vi "Update Method Event Unbundlers.vi"(8 "error in (no error)":errorcluster, 11 "VI ref in":refnum<vi>) -> (0 "error out":errorcluster, 2 "RPC Method Name":string, 3 "VI ref out":refnum<vi>)   [LabVIEW 2019, in "gRPC Scripting Tools.lvlib"]
uses:
  gRPC Scripting Tools.lvlib
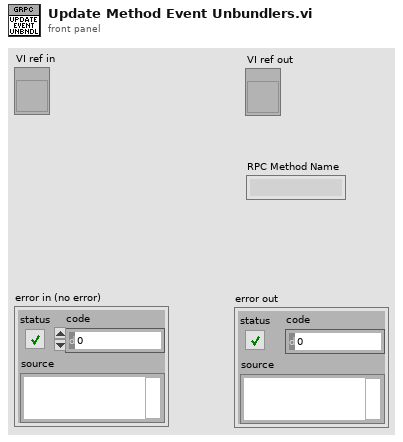
[diagram p1: front panel]
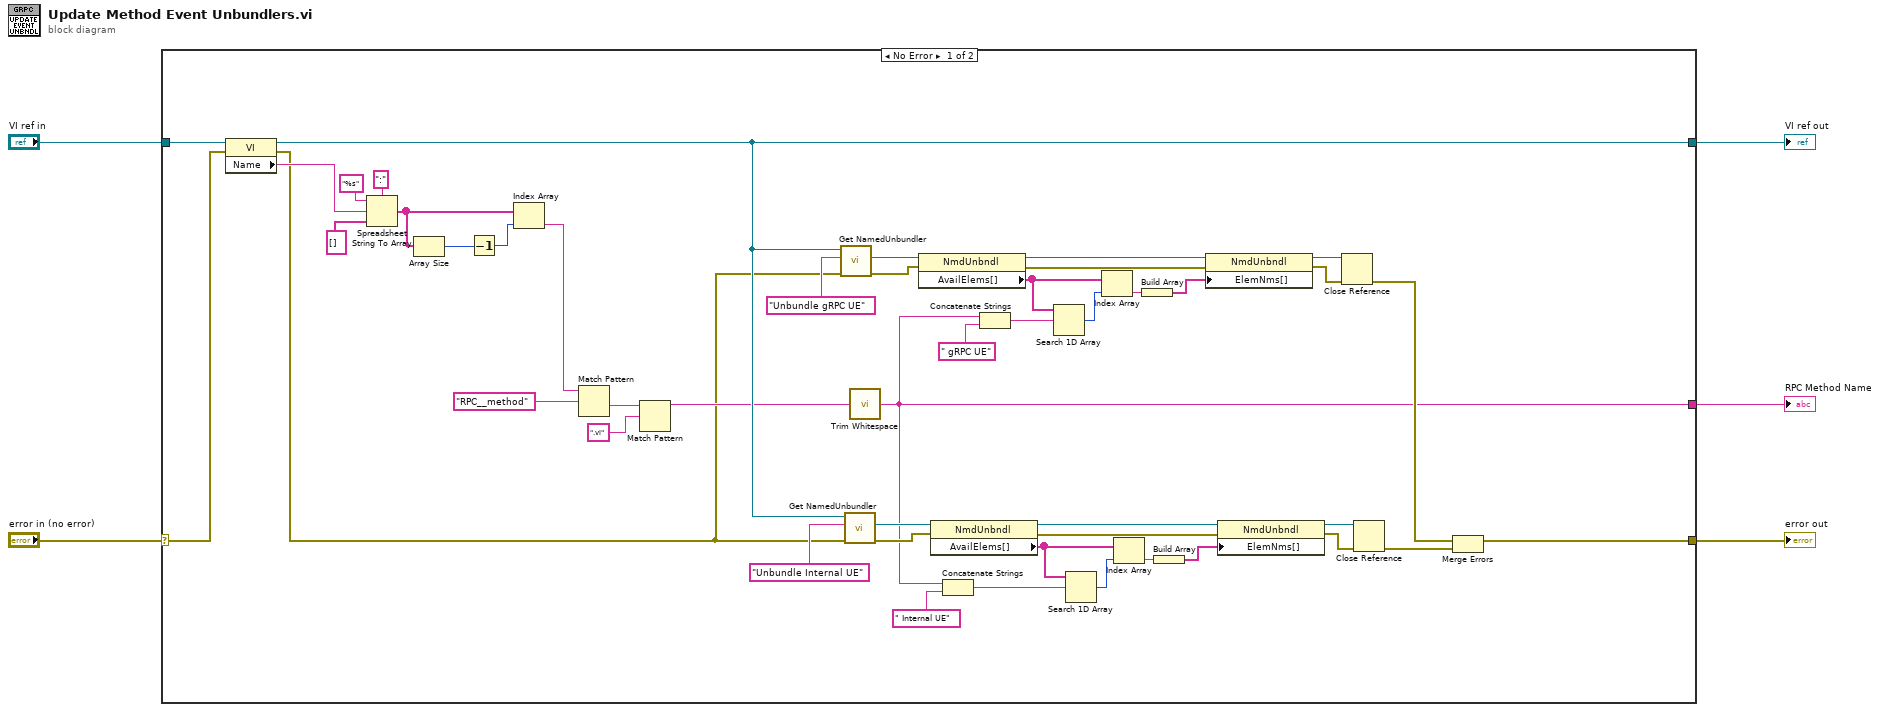
[diagram p0: block diagram]
diagram:
  n1 = case shown="No Error" "error in (no error)" {
    selector: "error in (no error)" -> [w8 w53]
    tunnel: [w51 w53] -> w5
    tunnel: "VI ref in" -> [w22 w52]
    tunnel: [w21 w52] -> w2
    tunnel: [w6 _] -> w1
    frame No Error {
      n2 = property class="VI"(reference=w22, error in=w8) -> (reference out=w21:refnum<vi>, error out=w7:errorcluster, "Name"=w19:string)
      n3 = Spreadsheet String To Array(delimiter (Tab)=":", format string="%s", spreadsheet string=w19, array type (2D Dbl)=string[] []) -> (array=w14:string[])
      n4 = Array Size(array=w14) -> (size(s)=w16:i32)
      n5 = Decrement(x=w16) -> (x-1=w15:i32)
      n6 = Index Array(array=w14, index=w15) -> (element=w11:string)
      n7 = Match Pattern(string=w11, regular expression="RPC__method") -> (after substring=w13:string)  [unwired: 1 in, 3 out]
      n8 = Match Pattern(string=w13, regular expression=".vi") -> (before substring=w10:string)  [unwired: 1 in, 3 out]
      n9 = call "Get NamedUnbundler.vi"("error in (no error)"=w7, "Label"="Unbundle gRPC UE" ("name/order"), "Owner VI in"=w21) -> ("error out"=w47:errorcluster, "NamedUnbundler ref out"=w24:refnum<vi>)  [unwired: 5 in, 2 out]
      n10 = call "Get NamedUnbundler.vi"("error in (no error)"=w7, "Label"="Unbundle Internal UE" ("name/order"), "Owner VI in"=w21) -> ("error out"=w48:errorcluster, "NamedUnbundler ref out"=w40:refnum<vi>)  [unwired: 5 in, 2 out]
      n11 = call <vilib>:"Trim Whitespace.vi"("string"=w10) -> ("trimmed string"=w6:string)  [unwired: 1 in]
      n12 = property class="NmdUnbndl"(reference=w24, error in=w47) -> (reference out=w29:refnum<vi>, error out=w32:errorcluster, "AvailElems[]"=w28:string[])
      n13 = property class="NmdUnbndl"(reference=w40, error in=w48) -> (reference out=w36:refnum<vi>, error out=w39:errorcluster, "AvailElems[]"=w35:string[])
      n14 = Concatenate Strings(w6, " Internal UE" ("string")) -> (w42:string)
      n15 = Concatenate Strings(w6, " gRPC UE" ("string")) -> (w26:string)
      n16 = Search 1D Array(1D array=w28, element=w26) -> (index of element=w27:i32)  [unwired: 1 in]
      n17 = Search 1D Array(1D array=w35, element=w42) -> (index of element=w34:i32)  [unwired: 1 in]
      n18 = Index Array(array=w28, index=w27) -> (element=w30:string)
      n19 = Index Array(array=w35, index=w34) -> (element=w37:string)
      n20 = Build Array(w30) -> (w31:string[])
      n21 = Build Array(w37) -> (w38:string[])
      n22 = property class="NmdUnbndl"(reference=w29, error in=w32, "ElemNms[]"=w31) -> (reference out=w46:refnum<vi>, error out=w45:errorcluster)
      n23 = property class="NmdUnbndl"(reference=w36, error in=w39, "ElemNms[]"=w38) -> (reference out=w44:refnum<vi>, error out=w43:errorcluster)
      n24 = Close Reference(reference=w46, error in (no error)=w45) -> (error out=w49:errorcluster)
      n25 = Close Reference(reference=w44, error in (no error)=w43) -> (error out=w50:errorcluster)
      n26 = Merge Errors(w49, w50) -> (w51:errorcluster)
    }
    frame Error {
    }
  }
  "error out" <- w5
  "VI ref out" <- w2
  "RPC Method Name" <- w1
